vi "getAngle.vi"(6 "Channel":i32, 8 "error in (no error)":errorcluster, 11 "Inst.Xeryon-Rotator in":refnum<class "Inst.Xeryon-Rotator.lvclass">) -> (0 "error out":errorcluster, 1 "Status":string, 2 "Angle (°)":dbl, 3 "Inst.Xeryon-Rotator out":refnum<class "Inst.Xeryon-Rotator.lvclass">, 4 "Finished?":bool)   [LabVIEW 2019, in "Inst.Xeryon-Rotator.lvclass"]
uses:
  Inst.Xeryon-Rotator.lvclass
  C:/Program Files (x86)/National Instruments/LabVIEW 2019/user.lib/LevyLab/Instrument Framework/Instrument/Instrument.lvclass
  Typedefs/Inst.Xeryon-Rotator.Commands--Enum.ctl
  <userlib>/LevyLab/Instrument Framework/Instrument Types/Cryostat/Typedefs/getAngle--cluster.ctl
  773e2a9d-0901-4956-ae6e-010e7225b876.vi
  773e2a9d-0901-4956-ae6e-010e7225b876.vi/11828800-3453-4f84-86bd-3e81b3592072.vi
  773e2a9d-0901-4956-ae6e-010e7225b876.vi/0ca54dff-c6eb-4130-ae76-37ac1b1013e3.vi
  <vilib>/Utility/Data Type/Get Type Information.vi
  <vilib>/JDP Science/JSONtext/JSON text to Variant.vi
  <vilib>/JDP Science/JSONtext/LVClass Serializer/JSONtext LVClass Serializer.lvclass
  <userlib>/LevyLab/Instrument Framework/Instrument/Instrument.lvclass
  <userlib>/LevyLab/Instrument Framework/Instrument Types/Cryostat/Instrument.Cryostat.lvclass
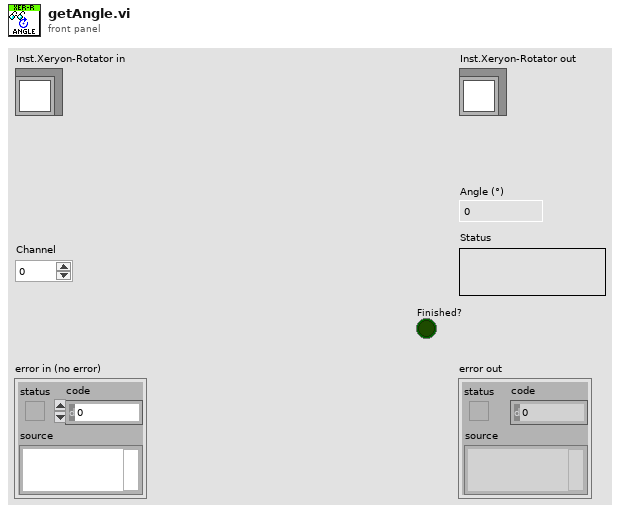
[diagram p1: front panel]
types:
  T1 = typedef "Instrument.Cryostat.lvclass/getAngle--cluster.ctl" = cluster{"angle":dbl, "status":string, "finished":bool}
  T2 = typedef "Inst.Xeryon-Rotator.lvclass/Inst.Xeryon-Rotator.Commands--Enum.ctl" = enum16{"setAngle", "getAngle", "setState"}
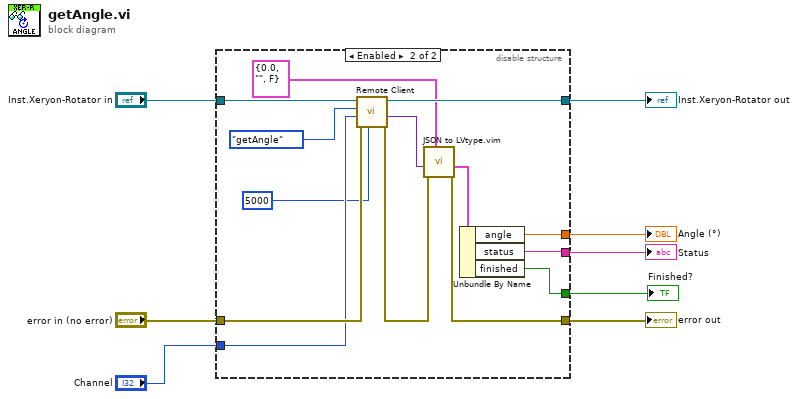
[diagram p0: block diagram]
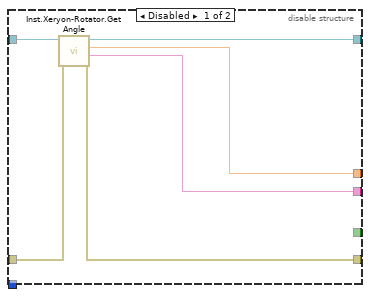
[diagram p2: hidden frame]
diagram:
  n1 = disable-structure shown="Enabled" {
    disable-tunnel: "Inst.Xeryon-Rotator in" -> [w14 w28]
    disable-tunnel: [w13 w27] -> w7
    disable-tunnel: [w12 w16] -> w6
    disable-tunnel: "error in (no error)" -> [w11 w23]
    disable-tunnel: [w10 w24] -> w4
    disable-tunnel: [w9 w25] -> w3
    disable-tunnel: "Channel" -> [_ w22]
    disable-tunnel: [_ w15] -> w1
    frame Disabled {
      n2 = call "Inst.Xeryon-Rotator.Get Angle.vi"("error in (no error)"=w11, "Inst.Xeryon-Rotator in"=w14) -> ("error out"=w12:errorcluster, "delimited string"=w10:string, "EPOS In Current Units"=w9:dbl, "Inst.Xeryon-Rotator out"=w13:refnum<class "Inst.Xeryon-Rotator.lvclass">)  [unwired: 6 in]
    }
    frame Enabled {
      n3 = call <userlib>:"Remote Client.vi"("timeout (ms) [500]"=5000, "error in (no error)"=w23, "Data in"=w22, "Command in"=Inst.Xeryon-Rotator.Commands--Enum."getAngle" ("Commands"), "Instrument in"=w28) -> ("error out"=w17:errorcluster, "Data out"=w19:variant, "Instrument out"=w27:refnum<class "Inst.Xeryon-Rotator.lvclass">)  [unwired: 3 in, 1 out]
      n4 = call "JSON to LVtype.vim"("type"=T1 {"angle"=0.0, "status"="", "finished"=FALSE} ("getAngle"), "error in (no error)"=w17, "JSON Data in"=w19) -> ("error out"=w16:errorcluster, "Data out"=w18:T1)  [unwired: 7 in]
      n5 = Unbundle By Name(w18) -> ("angle"=w25:dbl, "status"=w24:string, "finished"=w15:bool)
    }
  }
  "error out" <- w6
  "Inst.Xeryon-Rotator out" <- w7
  "Angle (°)" <- w3
  "Status" <- w4
  "Finished?" <- w1
